vi "Get Configuration Settings.vi"(8 "error in (no error)":errorcluster) -> (0 "error out":errorcluster, 3 "Acquisition and Logging Configuration":T1={"Data Rate (Hz)"=1.0, "Samples per Read"=0, "Number of Reads to Save"=0, "Data File Name"="", "TDMS Properties"=[], "Number of Channels"=4, "Channel Scale Array"=[0.0, 0.0, 0.0, 0.0], "Channel Names"=[], "Trigger - RMS Value"=0.0, "Trigger - Channel"=0, "Trigger - Time (Minute)"=0, "Enable RMS Trigger"=FALSE, "Enable Time Trigger"=FALSE, "Always Log"=FALSE})   [LabVIEW 2022 SP3]
uses:
  controls/Acquisition and Logging Configuration.ctl
  controls/TDMS Properties.ctl
  <vilib>/Utility/xml.llb/Read From XML File(string).vi
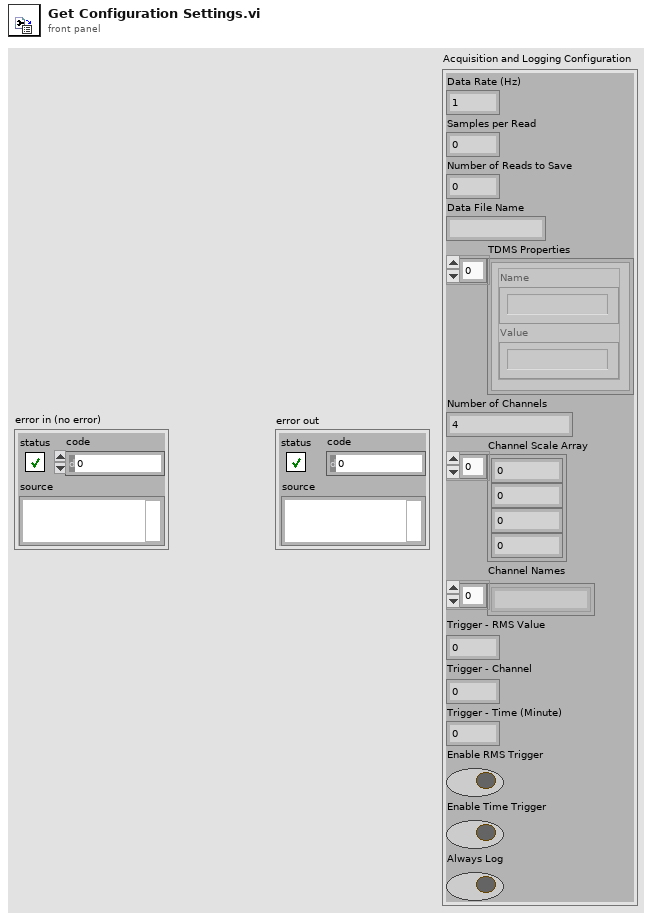
[diagram p1: front panel]
types:
  T1 = typedef "Acquisition and Logging Configuration.ctl" = cluster{"Data Rate (Hz)":dbl, "Samples per Read":i32, "Number of Reads to Save":i32, "Data File Name":string, "TDMS Properties":T2[], "Number of Channels":i32, "Channel Scale Array":dbl[], "Channel Names":string[], "Trigger - RMS Value":dbl, "Trigger - Channel":i32, "Trigger - Time (Minute)":i32, "Enable RMS Trigger":bool, "Enable Time Trigger":bool, "Always Log":bool}
  T2 = typedef "TDMS Properties.ctl" = cluster{"Name":string, "Value":string}
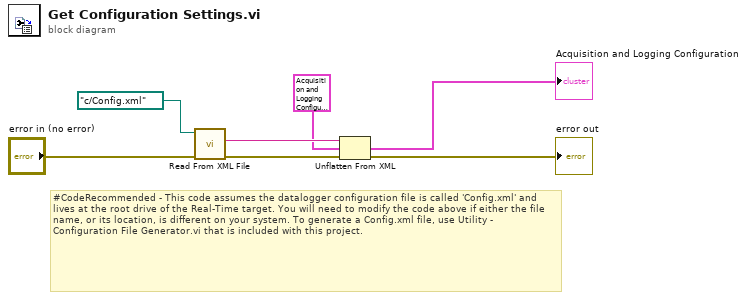
[diagram p0: block diagram]
diagram:
  # "#CodeRecommended - This code assumes the datalogger configuration file is called 'Config.xml' and lives at the root drive of the Real-Time target. You will need to modify the code above if either the file name, or its location, is different on your system. To generate a Config.xml file, use Utility - Configuration File Generator.vi that is included with this project."
  n1 = call-poly <vilib>:"Read From XML File.vi"("error in (no error)"="error in (no error)", "XML File Path"=path "c:/Config.xml") -> ("error out"=w6:errorcluster, "XML Elements"=w5:string)  [unwired: 7 in, 1 out]
  n2 = Unflatten From XML(xml string=w5, type=T1 {"Data Rate (Hz)"=0.0, "Samples per Read"=0, "Number of Reads to Save"=0, "Data File Name"="", "TDMS Properties"=[], "Number of Channels"=0, "Channel Scale Array"=[0.0, 0.0, 0.0, 0.0], "Channel Names"=[], "Trigger - RMS Value"=0.0, "Trigger - Channel"=0, "Trigger - Time (Minute)"=0, "Enable RMS Trigger"=FALSE, "Enable Time Trigger"=FALSE, "Always Log"=FALSE} ("VibLog Configuration"), error in (no error)=w6) -> (value=→"Acquisition and Logging Configuration":T1, error out=→"error out":errorcluster)
